vi "Wait_Seconds_with_display.vi"(2 "Message":string, 3 "Seconds to wait":dbl=1.0 format="%.2f") -> (1 "Stopped":bool)   [LabVIEW 2015]
doc: "Waits the number of seconds specified by the Seconds to Wait input, divided by the time dilation factor, if used."
uses:
  Globals/Meas_global.vi
panel:
  in  "stop":bool
  out "Seconds waited":u32(slide) scale=0.0..8.488436222076416
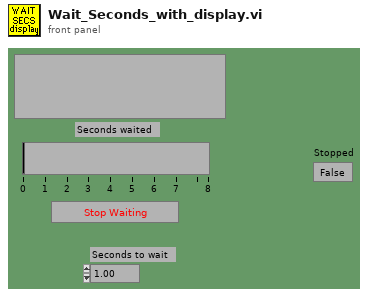
[diagram p1: front panel]
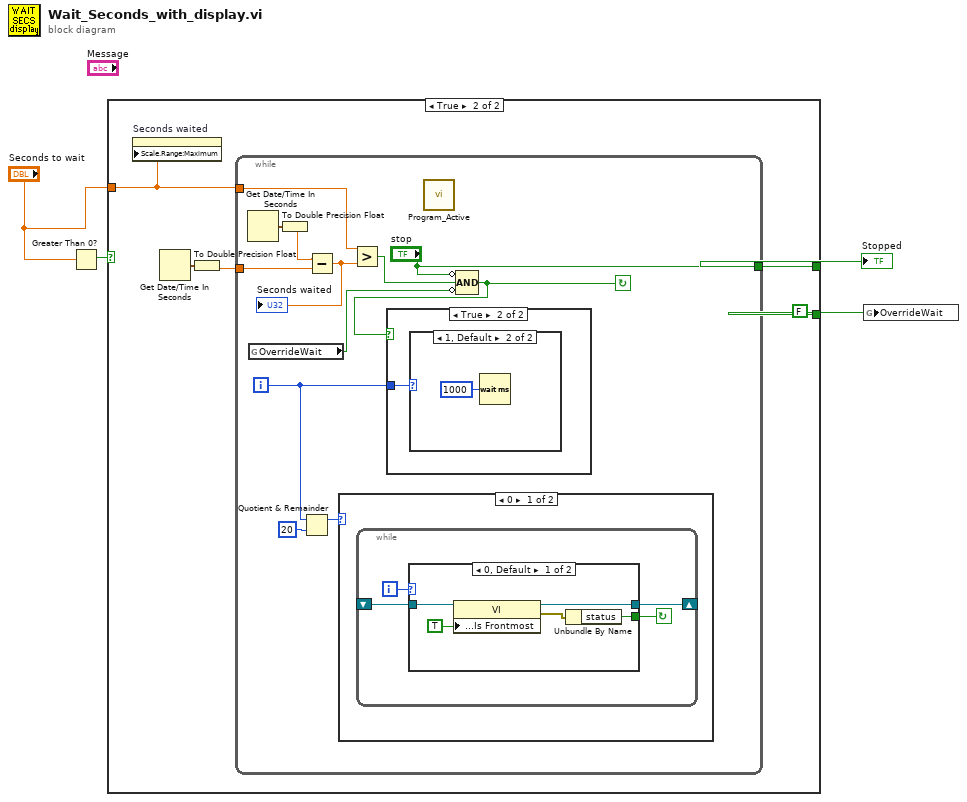
[diagram p0: block diagram]
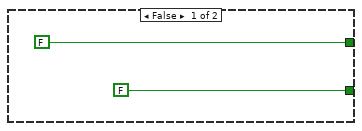
[diagram p2: hidden frame]
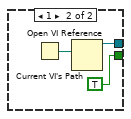
[diagram p3: hidden frame]
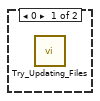
[diagram p6: hidden frame]
diagram:
  n1 = Greater Than 0?(x="Seconds to wait") -> (x > 0?=w3:bool)
  n2 = case shown="True" w3 {
    tunnel: [FALSE ("stop") w11] -> w4
    tunnel: "Seconds to wait" -> [_ w9]
    tunnel: [FALSE FALSE] -> w1
    frame False {
    }
    frame True {
      n3 = property on="Seconds waited" class="Slide (strict)"("Scale.Range:Maximum"=w9) -> ()  [unwired: 2 in, 2 out]
      n4 = Get Date/Time In Seconds() -> (seconds since 1Jan1904=w8:timestamp)
      n5 = To Double Precision Float(number=w8) -> (double precision float=w10:dbl)
      n6 = while {
        tunnel: ["stop"] -> w11
        tunnel: w9 -> [w20]
        tunnel: w10 -> [w23]
        i -> [w12]
        stop <- w16 continue-if-true
        n7 = Get Date/Time In Seconds() -> (seconds since 1Jan1904=w17:timestamp)
        n8 = global read "Meas_global.vi" "OverrideWait"() -> (w15:bool)
        n9 = To Double Precision Float(number=w17) -> (double precision float=w18:dbl)
        n10 = Quotient & Remainder(x=w12, y=20) -> (x-y*floor(x/y)=w14:i32)  [unwired: 1 out]
        n11 = Subtract(x=w18, y=w23) -> (x-y=w19:dbl)
        "Seconds waited" <- w19
        n12 = case shown="0" w14 {
          frame 0 {
            n13 = while {
              shift-left: _ -> [w27]
              shift-right: [w24] -> _
              i -> [w26]
              stop <- w25 continue-if-true
              n14 = case shown="0, Default" w26 {
                tunnel: w27 -> [w31 _]
                tunnel: [w29 TRUE ("status")] -> w25
                tunnel: [w28 w34] -> w24
                frame 0, Default {
                  n15 = property class="VI"(reference=w31, "Front Panel Window:Is Frontmost"=TRUE) -> (reference out=w28:refnum<vi>, error out=w30:errorcluster)  [unwired: 1 in]
                  n16 = Unbundle By Name(w30) -> ("status"=w29:bool)
                }
                frame 1 {
                  n17 = Current VI's Path() -> (path=w35:path)
                  n18 = Open VI Reference(vi path=w35) -> (vi reference=w34:refnum<vi>)  [unwired: 5 in, 1 out]
                }
              }
            }
          }
          frame 1, Default {
          }
        }
        n19 = Greater?(x=w20, y=w19) -> (0:w22:bool)
        n20 = call "Program_Active.vi"() -> ()  [unwired: 1 in]
        n21 = Compound Arithmetic op=AND(invert "stop", w22, invert w15) -> (w16:bool)
        n22 = case shown="True" w16 {
          tunnel: w12 -> [_ w36]
          frame False {
          }
          frame True {
            n23 = case shown="1, Default" w36 {
              frame 0 {
                n24 = call "Try_Updating_Files.vi"() -> ()  [unwired: 4 out]
              }
              frame 1, Default {
                n25 = Wait (ms)(milliseconds to wait=u32 1000) -> ()  [unwired: 1 out]
              }
            }
          }
        }
      }
    }
  }
  "Stopped" <- w4
  n26 = global write "Meas_global.vi" "OverrideWait"(w1) -> ()
